vi "FreeMemory.vi"(4 "Error IN Toolkit":i32, 5 "Error IN LabVIEW":errorcluster) -> (18 "Error OUT Toolkit":i32, 19 "Error OUT LabVIEW":errorcluster)   [LabVIEW 2018]
doc: "It free the two arrays stored in it during the processing from GPU memory.\n\nFor correct operation it should receive an error that comes from the VI \"CopyDataToCPU\"."
uses:
  dll/LibreriaAutis_3.dll
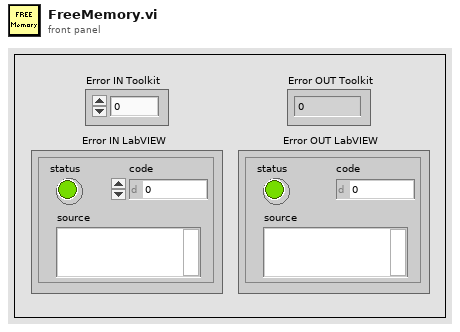
[diagram p1: front panel]
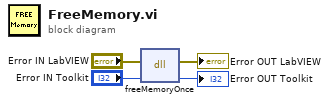
[diagram p0: block diagram]
diagram:
  n1 = dll-call lib="C:/Users/AUTIS/Desktop/LibreriaAUTIS/LabVIEW/dll/LibreriaAutis_3.dll" fn="freeMemoryOnce"(error in="Error IN LabVIEW", "error"="Error IN Toolkit") -> (error out=→"Error OUT LabVIEW":errorcluster, "error"=→"Error OUT Toolkit":i32)  [unwired: 3 in, 1 out]
